vi "refmgr_remove.vi"() -> ()   [LabVIEW 2014, in "RefManager(dev).lvlib"]
uses:
  RefManager(dev).lvlib
  <userlib>/_NEVSTOP/TagDB/Core/TagDB.lvlib
  <userlib>/_NEVSTOP/TagDB/Core/tagDB_Def.ctl
  <userlib>/_NEVSTOP/TagDB/Core/_Support/Properties/tagDB dbChanged.vi
  <userlib>/_NEVSTOP/TagDB/Core/_Support/Properties/tagDB getTags.vi
  <userlib>/_NEVSTOP/TagDB/Core/_Support/Access/_variant.vi
  <userlib>/_NEVSTOP/TagDB/Core/_Support/Error/_Clear Errors.vi
  <userlib>/_NEVSTOP/TagDB/Core/_XNode/tagDB_value.xnode/tagDB_value.xnode
panel:
  out "Keys":string[](array[string])
  out "References":refnum<vi>[](array[refnum])
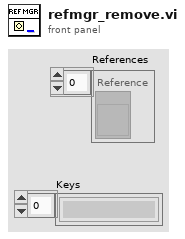
[diagram p1: front panel]
types:
  T1 = typedef "TagDB.lvlib/tagDB_Def.ctl" = refnum<k1>
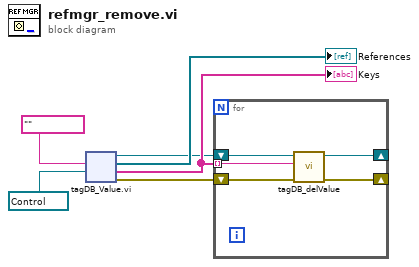
[diagram p0: block diagram]
diagram:
  n1 = xnode "tagDB_Value.vi"("Type"=refnum<vi> refnum, "RegExp"="") -> ("error out"=w1:errorcluster, "DB Ref(dup)"=w2:T1, "value"=→"References":refnum<vi>[], "names"=w4:string[])  [unwired: 2 in]
  "Keys" <- w4
  n2 = for {
    tunnel: w4 -> [w7] mode=indexing
    shift-right: [w10] -> _
    shift-left: w2 -> [w11]
    shift-right: [w9] -> _
    shift-left: w1 -> [w8]
    n3 = call <userlib>:"tagDB_delValue.vi"("error in (no error)"=w8, "name"=w7, "DB Ref"=w11) -> ("error in (no error) (dup)"=w9:errorcluster, "DB Ref (dup)"=w10:T1)  [unwired: 7 in]
  }
